vi "ST_parse_operator_data.vi"(6 "recordset_data":variant[][](array[variant]), 8 "error_in":errorcluster, 11 "command_nmb":u8) -> (0 "error_out":errorcluster, 3 "reference_data_to_PLC":u8[](array[numeric]))   [LabVIEW 2020]
uses:
  _misc/byte_array_parser/from_STR_to_PLC_STRING[50].vi
  <vilib>/addons/database/_DB Variant To Data/Database Variant To Data.xnode
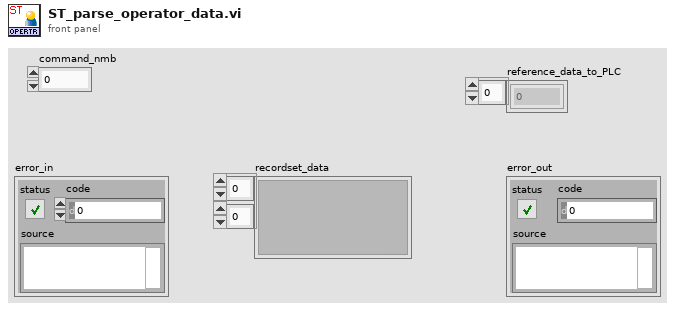
[diagram p1: front panel]
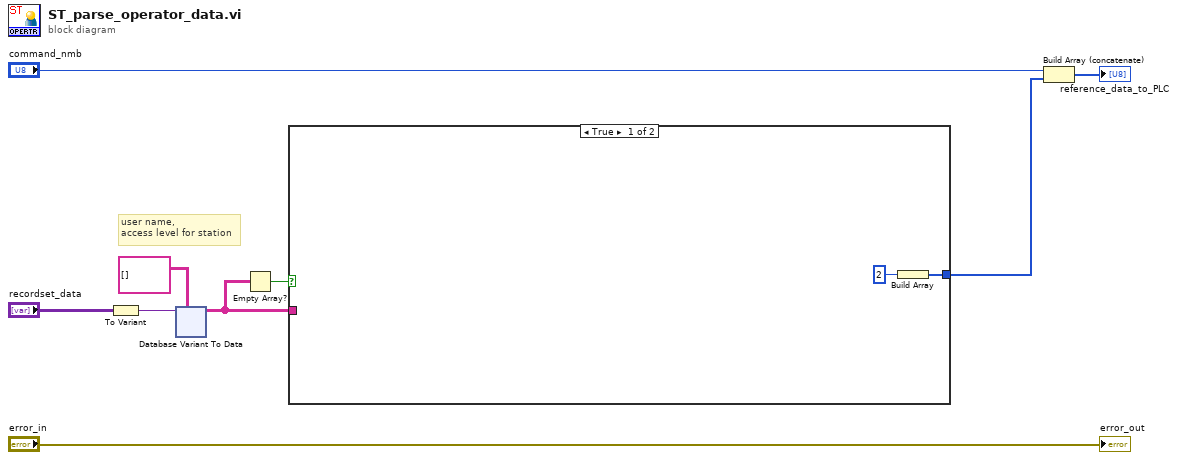
[diagram p0: block diagram]
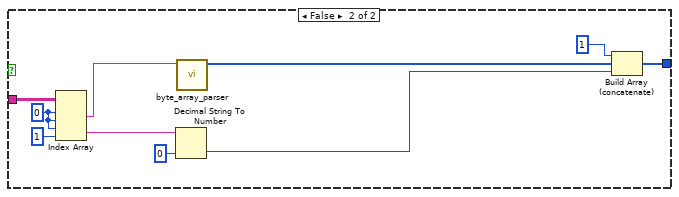
[diagram p2: hidden frame]
diagram:
  # "user name,\naccess level for station"
  n1 = To Variant(anything="recordset_data") -> (Variant=w5:variant)
  n2 = xnode "Database Variant To Data"("database variant"=w5, "type"=string[][] []) -> ("data"=w1:string[][])  [unwired: 1 in, 1 out]
  n3 = Empty Array?(array=w1) -> (empty?=w3:bool)
  n4 = case shown="True" w3 {
    tunnel: [w10 w14] -> w2
    tunnel: w1 -> [_ w21]
    frame True {
      n5 = Build Array(u8 2) -> (w10:u8[])
    }
    frame False {
      w20 = 0 ("index (row)")
      n6 = Index Array(array=w21, index (row) #1=w20, index (col) #1=w20, index (row) #2=w20, index (col) #2=1 ("disabled index (col)")) -> (element #1=w16:string, element #2=w18:string)
      n7 = Decimal String To Number(string=w18, default (0L)=u8 0 ("default (0 I32)")) -> (number=w13:u8)  [unwired: 1 in, 1 out]
      n8 = call-poly "byte_array_parser.vi"("String"=w16) -> ("byte_array"=w15:u8[])  [unwired: 9 in, 1 out]
      n9 = Build Array (concatenate)(u8 1, w15, w13) -> (w14:u8[])
    }
  }
  n10 = Build Array (concatenate)("command_nmb", w2) -> (→"reference_data_to_PLC":u8[])
  "error_out" <- "error_in"
